vi "LVClass_CorrectionDataManager SetInteractionMatrixPreferences.vi"(0 "CorrectionDataManager in":refnum<class "CorrectionDataManager.lvclass">, 5 "push_pull_value":T1, 11 "error in (no error)":errorcluster) -> (4 "CorrectionDataManager out":refnum<class "CorrectionDataManager.lvclass">, 15 "error out":errorcluster)   [LabVIEW 2020, in "CorrectionDataManager.lvclass"]
doc: "Calibration process supposes back and forth moves on all actuators.\n\n<B>corrdata_managerIn</B> : CorrDataManager object.\n<B>corrdata_managerOut</B> : CorrDataManager object.\n<B>push_pull_value</B> : In case experiment type is \"push-pull\" (type 0), indicates the actuators\n displacement amplitude."
uses:
  CorrectionDataManager.lvclass
  InteractionMatrixAcquisitionParameters.ctl
  LVClass_CorrectionDataManager Read CorrectionDataManager.vi
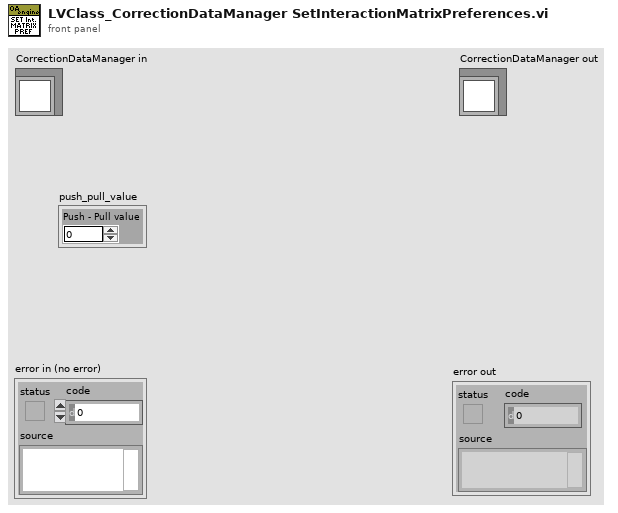
[diagram p1: front panel]
types:
  T1 = typedef "InteractionMatrixAcquisitionParameters.ctl" = cluster{"Push - Pull value":sgl}
  T2 = typedef "ClassID.ctl" = i64
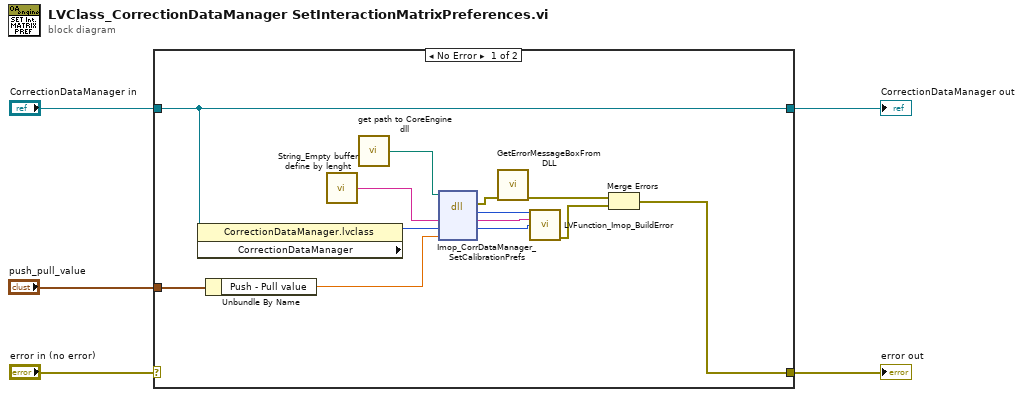
[diagram p0: block diagram]
diagram:
  n1 = case shown="No Error" "error in (no error)" {
    selector: "error in (no error)" -> [_ w20]
    tunnel: [w10 w20] -> w2
    tunnel: [w11 w19] -> w5
    tunnel: "CorrectionDataManager in" -> [w11 w19]
    tunnel: "push_pull_value" -> [w8 _]
    frame No Error {
      n2 = property class="CorrectionDataManager.lvclass"(reference=w11) -> ("CorrectionDataManager"=w9:T2)  [unwired: 1 in, 2 out]
      n3 = Unbundle By Name(w8) -> ("Push - Pull value"=w7:sgl)
      n4 = call "String_Empty buffer define by lenght.vi"() -> ("Empty buffer"=w16:string)  [unwired: 1 in]
      n5 = call "get path to CoreEngine dll.vi"() -> ("path to wavekit library"=w15:path)  [unwired: 14 in, 1 out]
      n6 = dll-call lib="D:/soft/HASO_v3/SVN_trunk/ImOpCoreEngine4_LV2011/DLLs/c_interface_vc100.dll" fn="Imop_CorrDataManager_SetCalibrationPrefs"(path in=w15, "message"=w16, "WavefrontCorrection"=w9, "push_pull_value"=w7) -> (error out=w14:errorcluster, "return type"=w18:i32, "message"=w17:string, "WavefrontCorrection"=w6:i64)  [unwired: 3 in, 1 out]
      n7 = call "GetErrorMessageBoxFromDLL.vi"("error IN"=w14) -> ("error OUT"=w13:errorcluster)  [unwired: 10 in]
      n8 = call "LVFunction_Imop_BuildError.vi"("code"=w18, "String to Prepend to source (\"\")"=w17, "Adresse"=w6) -> ("error out"=w12:errorcluster)  [unwired: 12 in]
      n9 = Merge Errors(w13, w12) -> (w10:errorcluster)
    }
    frame Error {
    }
  }
  "error out" <- w2
  "CorrectionDataManager out" <- w5
